vi "LAS-CTS_ControlProgram.vi"() -> ()   [LabVIEW 2024]
doc: "Shows how to move a motor to an absolute position."
uses:
  C:/Users/Behna/OneDrive/Documents/LAS/LAS-Labview-Controls/LAS LV Scan/Kinesis/Thorlabs.MotionControl.Controls.dll
  Kinesis/Thorlabs.MotionControl.Controls.dll
  <vilib>/Analysis/baseanly.llb/Mean (DBL).vi
  C:/Users/Behna/OneDrive/Documents/LAS/LAS-Labview-Controls/LAS LV Scan/Kinesis/ThorLabs.MotionControl.KCube.DCServoCLI.dll
  Kinesis/ThorLabs.MotionControl.KCube.DCServoCLI.dll
  <vilib>/Analysis/NI_AALBase.lvlib
  <vilib>/httpClient/LabVIEWHTTPClient.lvlib
panel:
  in  "Stop Laser":bool
  in  "Continuous Mode":bool
  in  "Rep Rate":u16(ring)=1 items=["20 Hz"=1, "10 Hz"=2, "5 Hz"=4, "4 Hz"=5, "2 Hz"=10, "1 Hz"=20]
  in  "Z position\n(Target mm)":dbl
  in  "X position\n(Target mm)":dbl
  in  "# of Pulses":i32
  out "E-meter Error":errorcluster
  in  "Fire Laser":bool
  in  "X Center (Mirror Coords)":dbl format="%.3g"
  in  "Z Center (Mirror Coords)":dbl format="%.3g"
  out "Filename":path
  in  "File #":i32 format="%03d"
  in  "base filename":string
  in  "Filepath":path
  in  "Target ID":string
  out "Laser Energy (uJ)":dbl format="%#.3f"
  out "Pulses Remaining":i32
  out "Laser \nOn/Off":bool
  in  "Energy Meter VISA port":refnum<visa-resource-name>="IntegraEnergyMeter"
  in  "KCubeDCServoControl Z axis":refnum<k24>(container)
  in  "KCubeDCServoControl X axis":refnum<k24>(container)
  out "CurrentPosZ(MC)":dbl=6.0
  out "CurrentPosX(MC)":dbl=6.0
  in  "SerialNumber Z":string="27261646"
  in  "SerialNumber X":string="27261828"
  # "Connection Setup"
  # "Laser Setup"
  # "ND Filter"
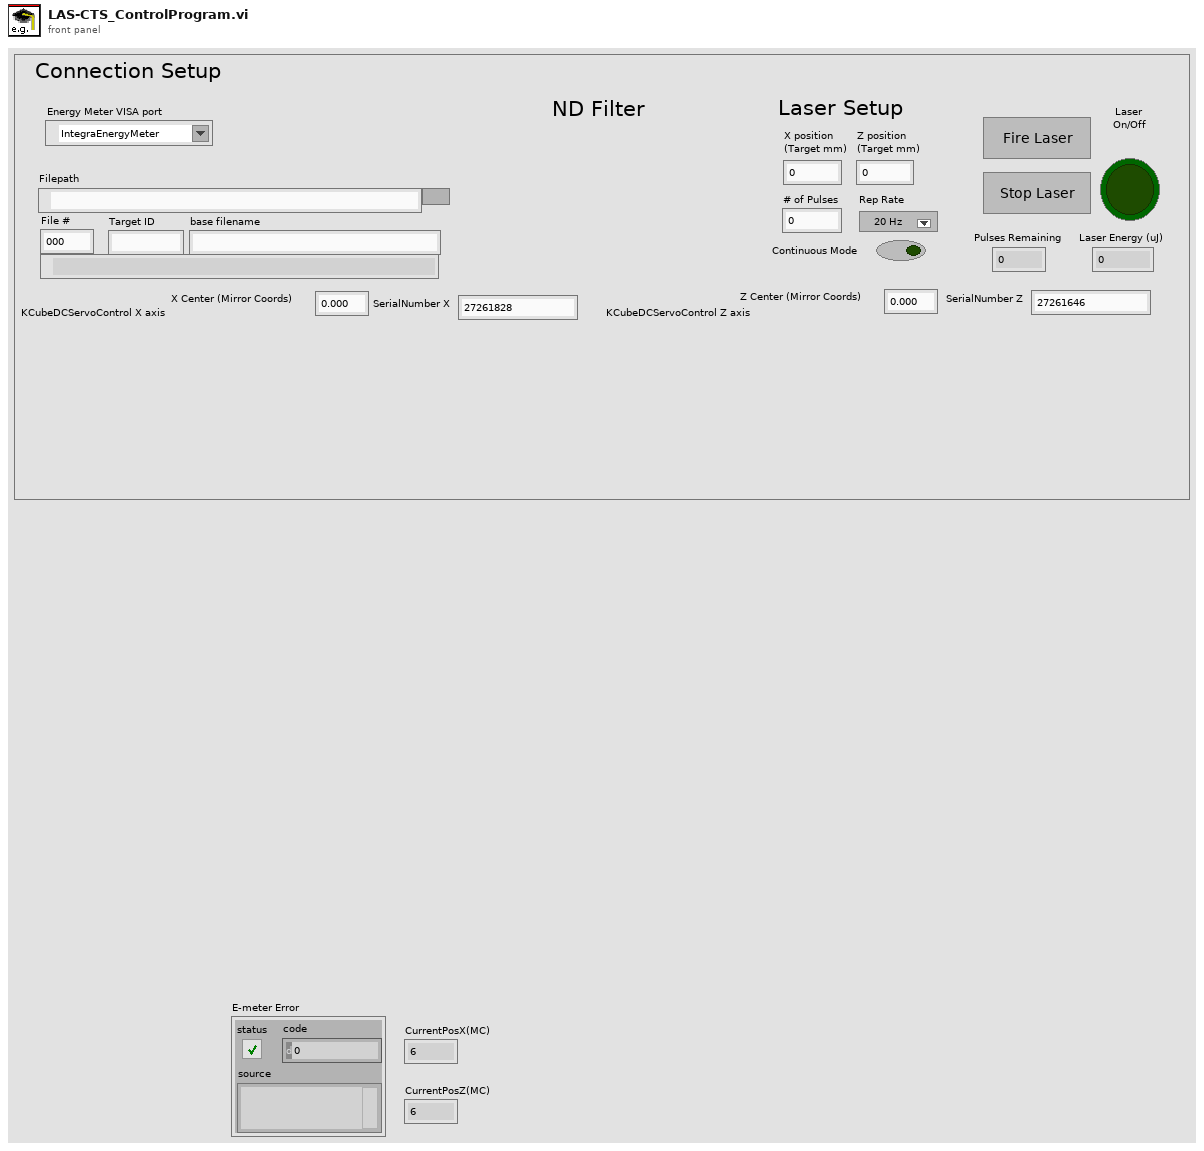
[diagram p1: front panel]
types:
  T1 = enum16{"open", "replace", "create", "open or create", "replace or create", "replace or create with confirmation"}
  T2 = typedef "LabVIEWHTTPClient.lvlib/ClientHandle.ctl" = refnum<k1>
  T3 = enum8{"Enabled", "Disabled", "Disabled and Grayed Out"}
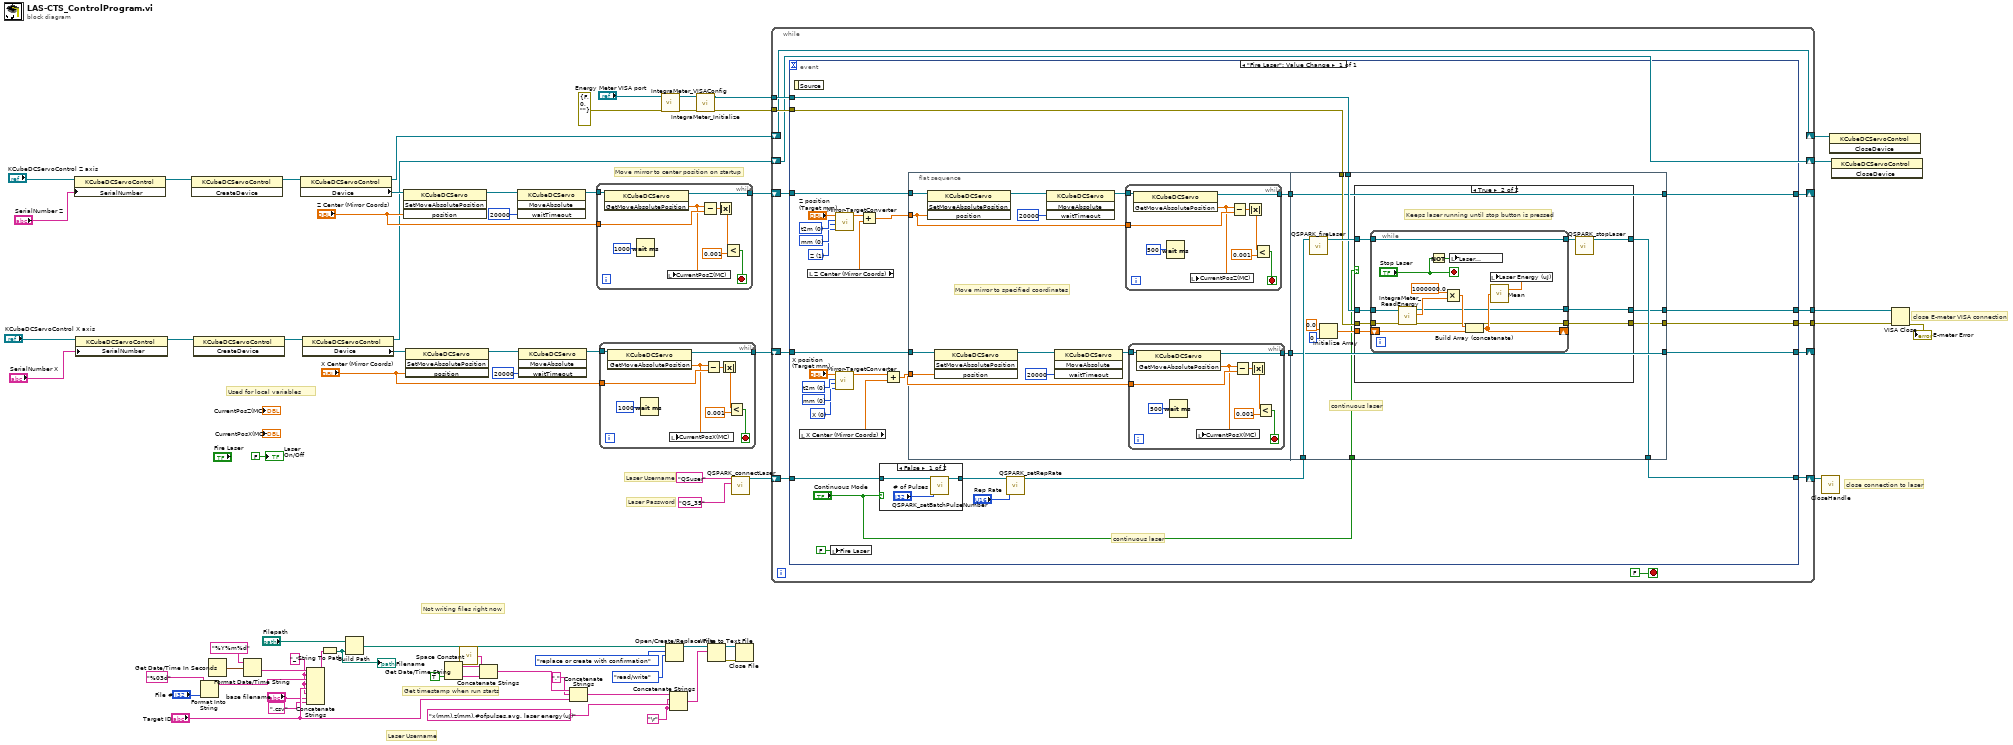
[diagram p0: block diagram]
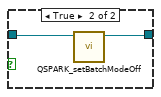
[diagram p2: hidden frame]
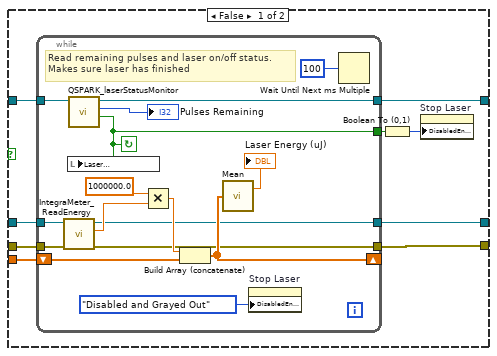
[diagram p3: hidden frame]
diagram:
  w27 = "_" ("string")
  w45 = "\r"
  # "Not writing files right now"
  # "close E-meter VISA connection"
  # "close connection to laser"
  # "Laser Username"
  # "Laser Password"
  # "Move mirror to center position on startup"
  # "Get timestamp when run starts"
  # "Used for local variables"
  # "Laser Username"
  n1 = property class="KCubeDCServoControl"(reference="KCubeDCServoControl Z axis", "SerialNumber"="SerialNumber Z") -> (reference out=w64:refnum<k24>)  [unwired: 1 in, 1 out]
  n2 = property class="KCubeDCServoControl"(reference="KCubeDCServoControl X axis", "SerialNumber"="SerialNumber X") -> (reference out=w67:refnum<k24>)  [unwired: 1 in, 1 out]
  n3 = invoke class="KCubeDCServoControl" method="CreateDevice"(reference=w64) -> (reference out=w60:refnum<k24>)  [unwired: 2 in, 2 out]
  n4 = invoke class="KCubeDCServoControl" method="CreateDevice"(reference=w67) -> (reference out=w65:refnum<k24>)  [unwired: 2 in, 2 out]
  n5 = Format Into String(format string="%03d", "File #") -> (resulting string=w30:string)  [unwired: 2 in, 1 out]
  n6 = Get Date/Time In Seconds() -> (seconds since 1Jan1904=w35:timestamp)
  n7 = Format Date/Time String(time format string (%c)="%Y%m%d", seconds (now)=w35) -> (date/time string=w33:string)  [unwired: 1 in]
  n8 = property class="KCubeDCServoControl"(reference=w60) -> (reference out=w10:refnum<k24>, "Device"=w22:refnum<k24>)  [unwired: 1 in, 1 out]
  n9 = property class="KCubeDCServoControl"(reference=w65) -> (reference out=w8:refnum<k24>, "Device"=w53:refnum<k24>)  [unwired: 1 in, 1 out]
  n10 = Concatenate Strings(w33, w27, w30, w27, "Target ID", w27, "base filename", ".csv" ("string")) -> (w36:string)
  n11 = String To Path(string=w36) -> (path=w24:path)
  "Filename" <- w24
  n12 = Build Path(base path="Filepath", name or relative path=w24) -> (appended path=w29:path)
  n13 = invoke class="KCubeDCServo" method="SetMoveAbsolutePosition"(reference=w22, "position"="Z Center (Mirror Coords)") -> (reference out=w57:refnum<k24>)  [unwired: 2 in, 3 out]
  n14 = invoke class="KCubeDCServo" method="SetMoveAbsolutePosition"(reference=w53, "position"="X Center (Mirror Coords)") -> (reference out=w55:refnum<k24>)  [unwired: 2 in, 3 out]
  n15 = Get Date/Time String(want seconds? (F)=TRUE) -> (date string=w44:string, time string=w43:string)  [unwired: 2 in]
  n16 = call <vilib>:"Space Constant.vi"() -> ("String"=w42:string)
  n17 = Concatenate Strings(w44, w42, w43) -> (w40:string)
  n18 = invoke class="KCubeDCServo" method="MoveAbsolute"(reference=w57, "waitTimeout"=20000) -> (reference out=w21:refnum<k24>)  [unwired: 2 in, 3 out]
  n19 = invoke class="KCubeDCServo" method="MoveAbsolute"(reference=w55, "waitTimeout"=20000) -> (reference out=w19:refnum<k24>)  [unwired: 2 in, 3 out]
  n20 = Concatenate Strings(w40, "," ("string"), "Target ID") -> (w38:string)
  n21 = while {
    tunnel: "Z Center (Mirror Coords)" -> [w74]
    tunnel: [w72] -> w17
    tunnel: w21 -> [w70]
    stop <- w75 stop-if-true
    n22 = invoke class="KCubeDCServo" method="GetMoveAbsolutePosition"(reference=w70) -> (reference out=w72:refnum<k24>, "GetMoveAbsolutePosition"=w68:dbl)  [unwired: 2 in, 1 out]
    n23 = Wait (ms)(milliseconds to wait=u32 1000) -> ()  [unwired: 1 out]
    n24 = local write "CurrentPosZ(MC)"(w68) -> ()
    n25 = Subtract(x=w68, y=w74) -> (x-y=w71:dbl)
    n26 = Absolute Value(x=w71) -> (abs(x)=w76:dbl)
    n27 = Less?(x=w76, y=0.001) -> (x < y?=w75:bool)
  }
  n28 = while {
    tunnel: "X Center (Mirror Coords)" -> [w83]
    tunnel: [w81] -> w16
    tunnel: w19 -> [w79]
    stop <- w84 stop-if-true
    n29 = invoke class="KCubeDCServo" method="GetMoveAbsolutePosition"(reference=w79) -> (reference out=w81:refnum<k24>, "GetMoveAbsolutePosition"=w77:dbl)  [unwired: 2 in, 1 out]
    n30 = Wait (ms)(milliseconds to wait=u32 1000) -> ()  [unwired: 1 out]
    n31 = local write "CurrentPosX(MC)"(w77) -> ()
    n32 = Subtract(x=w77, y=w83) -> (x-y=w80:dbl)
    n33 = Absolute Value(x=w80) -> (abs(x)=w85:dbl)
    n34 = Less?(x=w85, y=0.001) -> (x < y?=w84:bool)
  }
  n35 = call "IntegraMeter_VISAConfig.vi"("error in (no error)"=errorcluster {"status"=FALSE, "code"=0, "source"=""}, "VISA resource name"="Energy Meter VISA port") -> ("error out"=w47:errorcluster, "reference out"=w46:refnum<visa-resource-name>)  [unwired: 8 in]
  n36 = Open/Create/Replace File(file path (use dialog)=w29, operation (0:open)=T1."replace or create with confirmation", access (0:read/write)=enum16{"read/write", "read-only", "write-only"}."read/write") -> (refnum out=w61:refnum<file>)  [unwired: 3 in, 2 out]
  n37 = Concatenate Strings(w38, w45, "x(mm),z(mm),#ofpulses,avg. laser energy(uJ)", w45) -> (w58:string)
  n38 = call "IntegraMeter_Initialize.vi"("error in"=w47, "VISA resource name"=w46) -> ("error out"=w14:errorcluster, "VISA resource name out"=w15:refnum<visa-resource-name>)  [unwired: 8 in]
  n39 = Write to Text File(file (use dialog)=w61, text=w58) -> (refnum out=w5:refnum<file>, error out=w6:errorcluster)  [unwired: 2 in, 1 out]
  n40 = call "QSPARK_connectLaser.vi"("password"="QS_35", "username"="QSuser") -> ("client handle out"=w4:T2)  [unwired: 9 in]
  n41 = Close File(refnum=w5, error in=w6) -> ()  [unwired: 2 out]
  n42 = while {
    tunnel: w15 -> [w96]
    tunnel: w14 -> [w95]
    shift-right: [w94] -> _
    shift-left: w17 -> [w98]
    shift-right: [w93] -> _
    shift-left: w16 -> [w97]
    tunnel: [w92] -> w13
    tunnel: [w91] -> w12
    shift-right: [w90] -> w9
    shift-left: w10 -> [w90]
    shift-right: [w89] -> w7
    shift-left: w8 -> [w89]
    shift-right: [w86] -> w1
    shift-left: w4 -> [w87]
    stop <- FALSE stop-if-true
    n43 = event shown="[0] \"Fire Laser\": Value Change" {
      selector: _ -> [_]
      dyn-events: _ -> [_]
      timeout: _ -> [_]
      tunnel: w98 -> [w129]
      tunnel: w97 -> [w128]
      tunnel: w96 -> [w118]
      tunnel: w95 -> [w117]
      tunnel: [w115] -> w94
      tunnel: [w114] -> w93
      tunnel: [w112] -> w86
      tunnel: [w111] -> w92
      tunnel: [w110] -> w91
      tunnel: w87 -> [w109]
      event "Fire Laser": Value Change {
        w122 = u16 0 items=["X", "Z"] ("axis")
        w123 = u16 0 items=["mm", "um"] ("input units")
        w124 = u16 0 items=["t2m", "m2t"] ("Conversion")
        w125 = u16 1 items=["X", "Z"] ("axis")
        w126 = u16 0 items=["mm", "um"] ("input units")
        w127 = u16 0 items=["t2m", "m2t"] ("Conversion")
        # "continuous laser"
        n44 = event-data() -> ()  [unwired: 1 in, 1 out]
        n45 = local read "X Center (Mirror Coords)"() -> (w100:dbl)
        n46 = local read "Z Center (Mirror Coords)"() -> (w105:dbl)
        n47 = local write "Fire Laser"(FALSE ("Fire Laser")) -> ()
        n48 = call "Mirror-TargetConverter.vi"("axis"=w122, "input units"=w123, "Conversion"=w124, "input distance"="X position\n(Target mm)") -> ("output distance"=w101:dbl)  [unwired: 7 in]
        n49 = call "Mirror-TargetConverter.vi"("axis"=w125, "input units"=w126, "Conversion"=w127, "input distance"="Z position\n(Target mm)") -> ("output distance"=w106:dbl)  [unwired: 7 in]
        n50 = Add(x=w106, y=w105) -> (x+y=w104:dbl)
        n51 = case shown="False" "Continuous Mode" {
          tunnel: w109 -> [w131 w134]
          tunnel: [w130 w133] -> w108
          frame False {
            n52 = call "QSPARK_setBatchPulseNumber.vi"("Number of Pulses"="# of Pulses", "client handle"=w131) -> ("client handle out"=w130:T2)  [unwired: 9 in]
          }
          frame True {
            n53 = call "QSPARK_setBatchModeOff.vi"("client handle"=w134) -> ("client handle out"=w133:T2)  [unwired: 10 in]
          }
        }
        n54 = Add(x=w101, y=w100) -> (x+y=w102:dbl)
        n55 = flat-sequence {
          tunnel: w104 -> [w138]
          tunnel: w129 -> [w143]
          tunnel: w128 -> [w140]
          tunnel: w102 -> [w137]
          tunnel: [w136] -> w116
          tunnel: [w135] -> w113
          tunnel: w120 -> [w177]
          tunnel: w118 -> [w175]
          tunnel: w117 -> [w174]
          tunnel: w116 -> [w170]
          tunnel: [w170] -> w115
          tunnel: [w169] -> w114
          tunnel: w113 -> [w169]
          tunnel: [w168] -> w112
          tunnel: [w167] -> w111
          tunnel: [w166] -> w110
          tunnel: "Continuous Mode" -> [w165]
          frame #0 {
            # "Move mirror to specified coordinates"
            n56 = invoke class="KCubeDCServo" method="SetMoveAbsolutePosition"(reference=w143, "position"=w138) -> (reference out=w146:refnum<k24>)  [unwired: 2 in, 3 out]
            n57 = invoke class="KCubeDCServo" method="SetMoveAbsolutePosition"(reference=w140, "position"=w137) -> (reference out=w142:refnum<k24>)  [unwired: 2 in, 3 out]
            n58 = invoke class="KCubeDCServo" method="MoveAbsolute"(reference=w146, "waitTimeout"=20000) -> (reference out=w144:refnum<k24>)  [unwired: 2 in, 3 out]
            n59 = invoke class="KCubeDCServo" method="MoveAbsolute"(reference=w142, "waitTimeout"=20000) -> (reference out=w139:refnum<k24>)  [unwired: 2 in, 3 out]
            n60 = while {
              tunnel: w138 -> [w162]
              tunnel: [w160] -> w136
              tunnel: w144 -> [w158]
              stop <- w163 stop-if-true
              n61 = invoke class="KCubeDCServo" method="GetMoveAbsolutePosition"(reference=w158) -> (reference out=w160:refnum<k24>, "GetMoveAbsolutePosition"=w156:dbl)  [unwired: 2 in, 1 out]
              n62 = Wait (ms)(milliseconds to wait=u32 500) -> ()  [unwired: 1 out]
              n63 = local write "CurrentPosZ(MC)"(w156) -> ()
              n64 = Subtract(x=w156, y=w162) -> (x-y=w159:dbl)
              n65 = Absolute Value(x=w159) -> (abs(x)=w164:dbl)
              n66 = Less?(x=w164, y=0.001) -> (x < y?=w163:bool)
            }
            n67 = while {
              tunnel: w137 -> [w153]
              tunnel: [w151] -> w135
              tunnel: w139 -> [w149]
              stop <- w154 stop-if-true
              n68 = invoke class="KCubeDCServo" method="GetMoveAbsolutePosition"(reference=w149) -> (reference out=w151:refnum<k24>, "GetMoveAbsolutePosition"=w147:dbl)  [unwired: 2 in, 1 out]
              n69 = Wait (ms)(milliseconds to wait=u32 500) -> ()  [unwired: 1 out]
              n70 = local write "CurrentPosX(MC)"(w147) -> ()
              n71 = Subtract(x=w147, y=w153) -> (x-y=w150:dbl)
              n72 = Absolute Value(x=w150) -> (abs(x)=w155:dbl)
              n73 = Less?(x=w155, y=0.001) -> (x < y?=w154:bool)
            }
          }
          frame #1 {
            # "continuous laser"
            n74 = call "QSPARK_fireLaser.vi"("client handle"=w177) -> ("client handle out"=w176:T2)  [unwired: 10 in]
            n75 = Initialize Array(0.0 ("element"), 0 ("dimension size")) -> (w171:dbl[])
            n76 = case shown="True" w165 {
              tunnel: w176 -> [w186 w204]
              tunnel: w175 -> [w185 w210]
              tunnel: w174 -> [w184 w209]
              tunnel: w171 -> [w183 w208]
              tunnel: [w182 w205] -> w168
              tunnel: [w181 w207] -> w167
              tunnel: [w180 w206] -> w166
              frame False {
                n77 = while {
                  tunnel: w186 -> [w202]
                  tunnel: w185 -> [w197]
                  tunnel: w184 -> [w196]
                  shift-right: [w194] -> _
                  shift-left: w183 -> [w195]
                  tunnel: [w191] -> w182
                  tunnel: [w190] -> w181
                  tunnel: [w189] -> w180
                  tunnel: [w187] -> w179
                  stop <- w187 continue-if-true
                  # "Read remaining pulses and laser on/off status. \nMakes sure laser has finished"
                  n78 = call "IntegraMeter_ReadEnergy.vi"("error in (no error)"=w196, "VISA resource name"=w197) -> ("error out"=w189:errorcluster, "Laser Energy (J)"=w199:dbl, "VISA resource name out"=w190:refnum<visa-resource-name>)  [unwired: 7 in]
                  n79 = call "QSPARK_laserStatusMonitor.vi"("client handle"=w202) -> ("laser on?"=w187:bool, "remaining pulses"=→"Pulses Remaining":i32, "client handle out"=w191:T2)  [unwired: 8 in]
                  n80 = local write "Laser \nOn/Off"(w187) -> ()
                  n81 = Multiply(x=1000000.0, y=w199) -> (x*y=w198:dbl)
                  n82 = Build Array (concatenate)(w198, w195) -> (w194:dbl[])
                  n83 = call-poly <vilib>:"Mean.vi"("X"=w194) -> ("mean"=→"Laser Energy (uJ)":dbl)  [unwired: 1 out]
                  n84 = property on="Stop Laser" class="Bool"("DisabledEnum"=T3."Disabled and Grayed Out" ("Disabled")) -> ()  [unwired: 2 in, 2 out]
                  n85 = Wait Until Next ms Multiple(millisecond multiple=u32 100) -> ()  [unwired: 1 out]
                }
                n86 = Boolean To (0,1)(Boolean=w179) -> (0, 1=w178:i16)
                n87 = property on="Stop Laser" class="Bool"("DisabledEnum"=w178) -> ()  [unwired: 2 in, 2 out]
              }
              frame True {
                # "Keeps laser running until stop button is pressed"
                n88 = while {
                  tunnel: w210 -> [w220]
                  tunnel: w209 -> [w219]
                  shift-right: [w217] -> _
                  shift-left: w208 -> [w218]
                  tunnel: [w214] -> w207
                  tunnel: [w213] -> w206
                  tunnel: w204 -> [w212]
                  tunnel: [w212] -> w203
                  stop <- "Stop Laser" stop-if-true
                  n89 = call "IntegraMeter_ReadEnergy.vi"("error in (no error)"=w219, "VISA resource name"=w220) -> ("error out"=w213:errorcluster, "Laser Energy (J)"=w222:dbl, "VISA resource name out"=w214:refnum<visa-resource-name>)  [unwired: 7 in]
                  n90 = Not(x="Stop Laser") -> (.not. x?=w215:bool)
                  n91 = Multiply(x=1000000.0, y=w222) -> (x*y=w221:dbl)
                  n92 = local write "Laser \nOn/Off"(w215) -> ()
                  n93 = Build Array (concatenate)(w221, w218) -> (w217:dbl[])
                  n94 = call-poly <vilib>:"Mean.vi"("X"=w217) -> ("mean"=w216:dbl)  [unwired: 1 out]
                  n95 = local write "Laser Energy (uJ)"(w216) -> ()
                }
                n96 = call "QSPARK_stopLaser.vi"("client handle"=w203) -> ("client handle out"=w205:T2)  [unwired: 10 in]
              }
            }
          }
        }
        n97 = call "QSPARK_setRepRate.vi"("Rep Rate"="Rep Rate", "client handle"=w108) -> ("client handle out"=w120:T2)  [unwired: 9 in]
      }
    }
  }
  n98 = call <vilib>:"CloseHandle.vi"("client handle"=w1) -> ()  [unwired: 14 in, 1 out]
  n99 = invoke class="KCubeDCServoControl" method="CloseDevice"(reference=w9) -> ()  [unwired: 2 in, 3 out]
  n100 = invoke class="KCubeDCServoControl" method="CloseDevice"(reference=w7) -> ()  [unwired: 2 in, 3 out]
  n101 = VISA Close(VISA resource name=w13, error in (no error)=w12) -> (error out=→"E-meter Error":errorcluster)
  "Laser \nOn/Off" <- FALSE ("Laser On/Off")
